vi "Shell Bundle Loss.vi"(6 "Mass Flux (kg/s-m^2)":dbl, 9 "Density (kg/m^3)":dbl, 10 "Friction Factor":dbl, 11 "Number Tube Rows":dbl) -> (3 "Bundle Loss (Pa)":dbl)   [LabVIEW 2019]
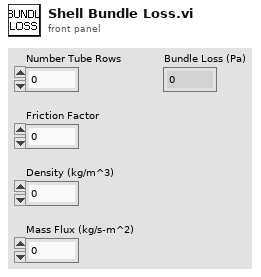
[diagram p1: front panel]
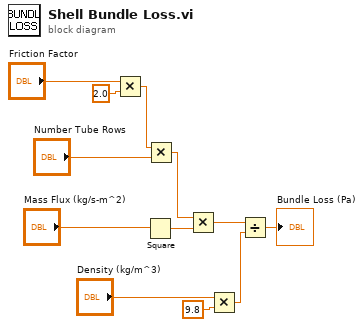
[diagram p0: block diagram]
diagram:
  n1 = Multiply(x="Friction Factor", y=2.0) -> (x*y=w4:dbl)
  n2 = Square(x="Mass Flux (kg/s-m^2)") -> (x^2=w5:dbl)
  n3 = Multiply(x=w4, y="Number Tube Rows") -> (x*y=w6:dbl)
  n4 = Multiply(x=w6, y=w5) -> (x*y=w8:dbl)
  n5 = Multiply(x="Density (kg/m^3)", y=9.8) -> (x*y=w11:dbl)
  n6 = Divide(x=w8, y=w11) -> (x/y=→"Bundle Loss (Pa)":dbl)
